vi "Begin.vi"(8 "error in":errorcluster) -> (0 "error out":errorcluster)   [LabVIEW 2019]
doc: "Called before other user functions, this VI is expected to open initial I/O refnums, load in file data, and do all program initialization. Notice that the <B>error out</B> terminal is simply used for data flow. Wiring it to other structures or subVIs ensures that this VI runs first."
uses:
  <vilib>/Rock Robotics/WPI/Joystick/WPI_JoystickDeviceEnum.ctl
  <vilib>/Rock Robotics/Network Tables/NT Write String Array.vi
  Robot Global Data.vi
  <vilib>/Rock Robotics/WPI/DriverStation/WPI_DriverStationRobotMode2.ctl
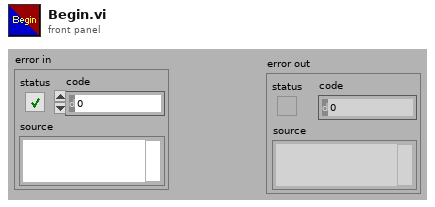
[diagram p1: front panel]
types:
  T1 = typedef "WPI_DriverStationRobotMode2.ctl" = enum16{"Autonomous Disabled", "Autonomous Enabled", "Teleop Disabled", "Teleop Enabled", "Disconnected", "Finish", "Test Disabled", "Test Enabled", "Emergency Stopped"}
  T2 = typedef "WPI_JoystickDeviceEnum.ctl" = enum16{"USB 0", "USB 1", "USB 2", "USB 3", "USB 4", "USB 5"}
  T3 = typedef "CTRE_CANifier_PWMChannel.ctl" = enum16{"PWMChannel0", "PWMChannel1", "PWMChannel2", "PWMChannel3"}
  T4 = typedef "CTRE_CANifier_DeviceRef.ctl" = cluster{"DeviceStatus":errorcluster, "Device Number":u8, "Handle":u64, "UsageFrame":u32, "Library Path":path}
  T5 = typedef "WPI_JoystickDevRef.ctl" = cluster{"Device":T2}
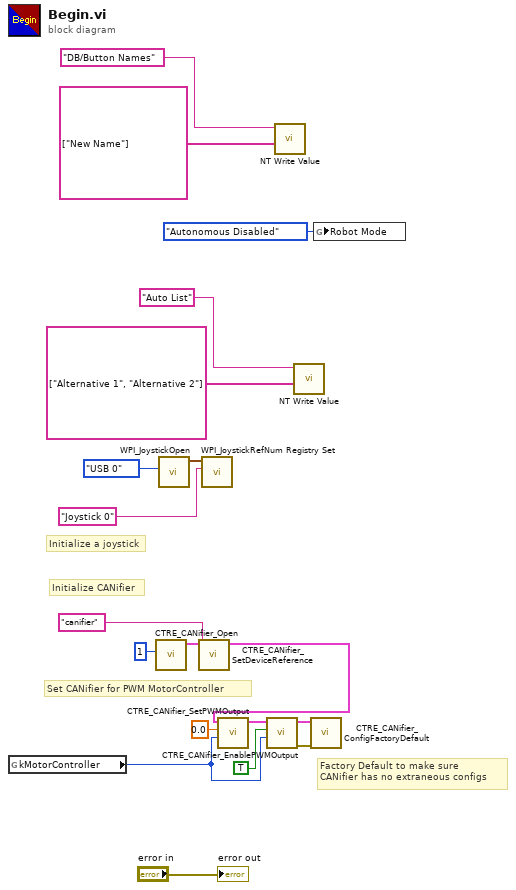
[diagram p0: block diagram]
diagram:
  # "Initialize a joystick"
  # "Factory Default to make sure\nCANifier has no extraneous configs"
  # "Set CANifier for PWM MotorController"
  # "Initialize CANifier"
  n1 = global read "Robot Global Data.vi" "kMotorController"() -> (w4:T3)
  n2 = call <vilib>:"CTRE_CANifier_Open.vi"("Device Number"=u8 1) -> ("CANifierDevRef"=w18:T4)  [unwired: 9 in, 1 out]
  n3 = call <vilib>:"WPI_JoystickOpen.vi"("JoystickDevice"=WPI_JoystickDeviceEnum."USB 0") -> ("JoystickDevRef"=w8:T5)  [unwired: 10 in]
  n4 = call <vilib>:"CTRE_CANifier_SetDeviceReference.vi"("refnum name"="canifier", "CANifierDevRef"=w18) -> ("CANifierDevRef"=w14:T4)  [unwired: 8 in, 1 out]
  n5 = call <vilib>:"WPI_JoystickRefNum Registry Set.vi"("refnum name"="Joystick 0", "JoystickDevRef"=w8) -> ()  [unwired: 8 in, 2 out]
  n6 = call <vilib>:"CTRE_CANifier_SetPWMOutput.vi"("PWMChannel"=w4, "Duty Cycle"=0.0, "CANifierDevRef"=w14) -> ("CANifierDevRef"=w15:T4)  [unwired: 7 in, 1 out]
  n7 = call <vilib>:"CTRE_CANifier_EnablePWMOutput.vi"("PWMChannel"=w4, "Enable?"=TRUE, "CANifierDevRef"=w15) -> ("error out"=w11:errorcluster, "CANifierDevRef"=w10:T4)  [unwired: 7 in]
  n8 = call-poly <vilib>:"NT Write Value.vi"("String Array"=string[] ["New Name"], "Name"="DB/Button Names") -> ()  [unwired: 9 in, 1 out]
  n9 = call-poly <vilib>:"NT Write Value.vi"("String Array"=string[] ["Alternative 1", "Alternative 2"], "Name"="Auto List") -> ()  [unwired: 9 in, 1 out]
  n10 = call <vilib>:"CTRE_CANifier_ConfigFactoryDefault.vi"("error in"=w11, "CANifierDevRef"=w10) -> ()  [unwired: 8 in, 2 out]
  n11 = global write "Robot Global Data.vi" "Robot Mode"(WPI_DriverStationRobotMode2."Autonomous Disabled" ("Robot Mode")) -> ()
  "error out" <- "error in"
